vi "CS POLARIS BME DG.Error2XMLFlatted call cluster.vi"(8 "call cluster in":T2, 10 "byteArray in":T1, 11 "error in":errorcluster) -> (0 "call cluster out":T2, 3 "error out":errorcluster)   [LabVIEW 2009, in "CS POLARIS BME DG.lvlib"]
uses:
  CS POLARIS BME DG.lvlib
  CSCore/CSSystem/CoreDefs/CoreDefs.call_type.ctl
  CSCore/BaseProcess/BaseProcess.descriptor string definition.ctl
  CSCore/CSSystem/CoreDefs/CoreDefs.rawDataType.ctl
  CSCore/CSSystem/CoreLib/CoreLib.string 2 byte array.vi
  CSCore/CSSystem/CoreLib/CoreLib.lvlib
  CSCore/BaseProcess/BaseProcess.lvlib
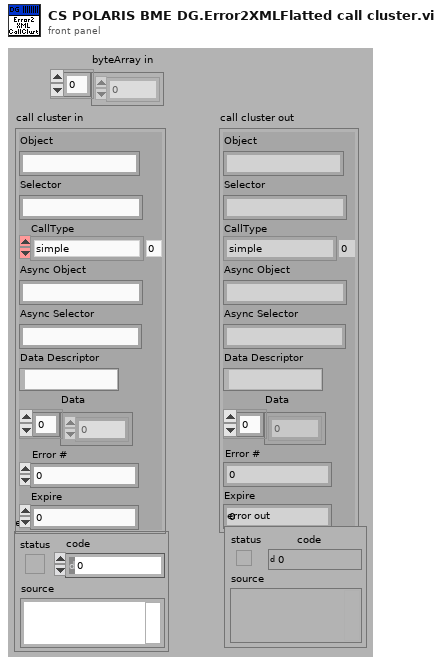
[diagram p1: front panel]
types:
  T1 = typedef "CoreDefs.rawDataType.ctl" = i8[]
  T2 = typedef "CoreDefs.call_type.ctl" = cluster{"Object":string, "Selector":string, "CallType":enum16{"simple", "synchronous", "asynchronous"}, "Async Object":string, "Async Selector":string, "Data Descriptor":T3, "Data":T1, "Error #":i32, "Expire":u32}
  T3 = typedef "BaseProcess.lvlib/BaseProcess.descriptor string definition.ctl" = string
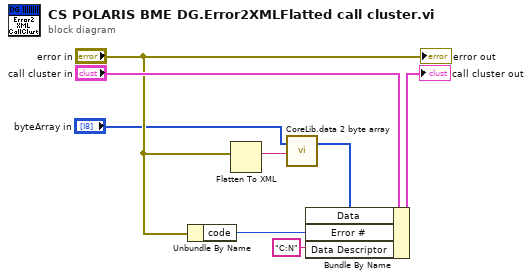
[diagram p0: block diagram]
diagram:
  n1 = Unbundle By Name("error in") -> ("code"=w4:i32)
  n2 = Flatten To XML(anything="error in") -> (xml string=w2:string)
  n3 = call-poly "CoreLib.data 2 byte array.vi"("byteArray"="byteArray in", "string"=w2) -> ("byteArray out"=w7:T1)  [unwired: 17 in]
  n4 = Bundle By Name(cluster="call cluster in", "Data"=w7, "Error #"=w4, "Data Descriptor"="C:N") -> (→"call cluster out":T2)
  "error out" <- "error in"
